vi "nirviLoopTimer.vi"(1 "Count(Ticks)":u32) -> (0 "Tick Count(Ticks)":u32)   [LabVIEW 2020]
doc: "Waits the value you specify in <B>Count</B> between loop iterations. You can call this function in a loop to control the loop execution rate. If an execution instance is missed, such as when the logic in the loop takes longer to execute than the specified interval, the Loop Timer Express VI returns immediately and establishes a new reference time stamp for subsequent calls. To manage execution rates with the Loop Timer Express VI, place the Loop Timer Express VI in the first frame of a Flat Sequence structure or a Stacked Sequence structure and put the rest of the code in subsequent frames."
panel:
  in  "Counter Units":u16(ring) items=["Ticks", "µSec", "mSec"]
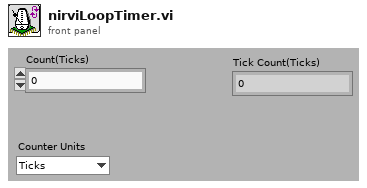
[diagram p1: front panel]
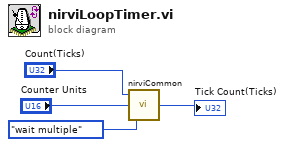
[diagram p0: block diagram]
diagram:
  n1 = call <vilib>:"nirviCommon.vi"("Action"=enum16{"wait", "wait multiple", "tick count"}."wait multiple", "Counter Units"="Counter Units", "Count(uSec)"="Count(Ticks)") -> ("Tick Count(uSec)"=→"Tick Count(Ticks)":u32)
